vi "ScanAction.vi"(8 "error in (no error)":errorcluster caption="entrée d'erreur (pas d'erreur)", 9 "IndicePoint":i32, 10 "Dir":bool, 11 "Monospec In":refnum<class "Monospec50.lvclass"> caption="DNL_LabVIEW Object in") -> (0 "error out":errorcluster caption="sortie d'erreur", 2 "ScanParsOut":dbl[](array[numeric]), 3 "Monospec Out":refnum<class "Monospec50.lvclass"> caption="DNL_LabVIEW Object out")   [LabVIEW 2019, in "Monospec50.lvclass"]
uses:
  Monospec50.lvclass
  C:/Programmes Labview/LabScanV1A/DevicesClass/BaseDevice/BaseDevice.lvclass
  Monospec50.lvclass/Monospec50.ctl
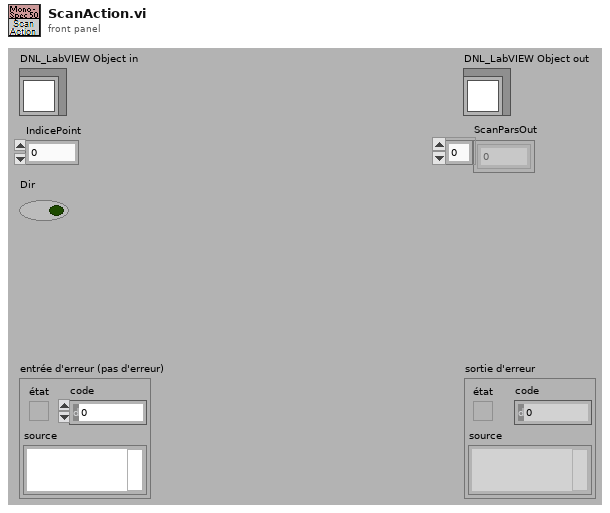
[diagram p1: front panel]
types:
  T1 = typedef "Monospec50.lvclass/Monospec50_Func.ctl" = enum16{"Position (nm)"}
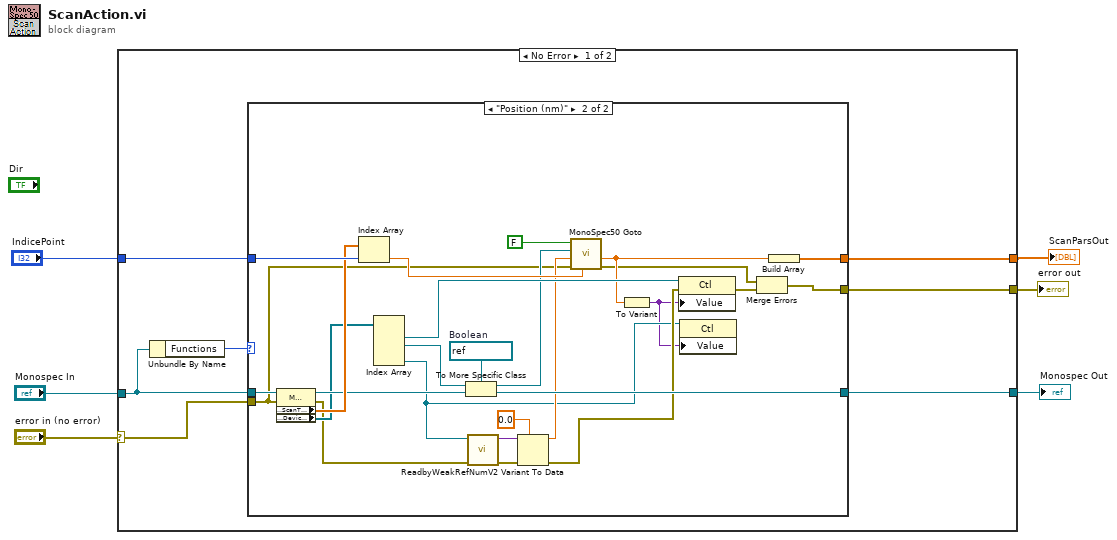
[diagram p0: block diagram]
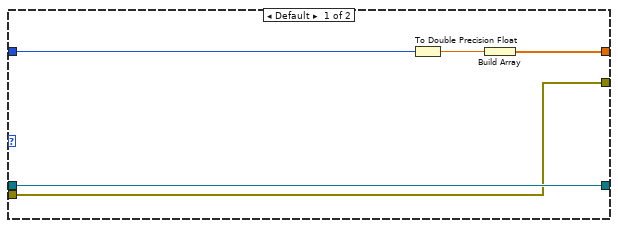
[diagram p2: hidden frame]
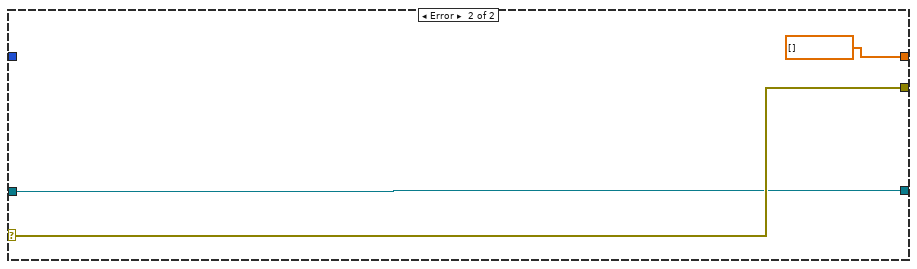
[diagram p3: hidden frame]
diagram:
  n1 = case shown="No Error" "error in (no error)" {
    selector: "error in (no error)" -> [w10 w46]
    tunnel: "Monospec In" -> [w11 w45]
    tunnel: [w9 dbl[] []] -> w1
    tunnel: [w8 w46] -> w4
    tunnel: [w7 w45] -> w3
    tunnel: "IndicePoint" -> [w12 _]
    frame No Error {
      n2 = Unbundle By Name(w11) -> ("Functions"=w13:T1)
      n3 = case shown="\"Position (nm)\"" w13 {
        tunnel: [w14 w43] -> w9
        tunnel: w12 -> [w18 w42]
        tunnel: [w16 w38] -> w7
        tunnel: w11 -> [w16 w40]
        tunnel: w10 -> [w15 w25]
        tunnel: [w15 w24] -> w8
        frame Default {
          n4 = To Double Precision Float(number=w18) -> (double precision float=w17:dbl)
          n5 = Build Array(w17) -> (w14:dbl[])
        }
        frame "Position (nm)" {
          w35 = refnum<vi> refnum  # Boolean
          n6 = property class="Monospec50.lvclass"(reference=w40, error in=w25) -> (reference out=w38:refnum<class "Monospec50.lvclass">, error out=w26:errorcluster, "Accessor:ScanTable"=w39:dbl[], "Accessor:DeviceCtrl"=w36:refnum<vi>[])
          n7 = Index Array(array=w39, index=w42) -> (element=w41:dbl)
          n8 = Index Array(array=w36) -> (element #1=w34:refnum<vi>, element #2=w32:refnum<vi>, element #4=w20:refnum<vi>)  [unwired: 4 in, 1 out]
          n9 = To More Specific Class(target class=w35, reference=w32) -> (specific class reference=w31:refnum<vi>)  [unwired: 1 in, 1 out]
          n10 = call <userlib>:"ReadbyWeakRefNumV2.vi"("error in"=w26, "Control Ref"=w20) -> ("error out"=w27:errorcluster, "Valeur"=w30:variant)  [unwired: 8 in]
          n11 = Variant To Data(error in=w27, type=0.0 ("PosAct"), Variant=w30) -> (data=w28:dbl, error out=w21:errorcluster)
          n12 = call <userlib>:"MonoSpec50 Goto.vi"("PosDem"=w41, "error in (no error)"=w25, "PosAct"=w28, "Moving Ref"=w31, "Ask Act Pos"=FALSE) -> ("error out"=w23:errorcluster, "PosAct Out"=w33:dbl)  [unwired: 3 in]
          n13 = To Variant(anything=w33) -> (Variant=w19:variant)
          n14 = property class="Ctl"(reference=w34, error in=w21, "Value"=w19) -> (error out=w22:errorcluster)  [unwired: 1 out]
          n15 = property class="Ctl"(reference=w20, "Value"=w19) -> ()  [unwired: 1 in, 2 out]
          n16 = Merge Errors(w23, w22) -> (w24:errorcluster)
          n17 = Build Array(w33) -> (w43:dbl[])
        }
      }
    }
    frame Error {
    }
  }
  "error out" <- w4
  "Monospec Out" <- w3
  "ScanParsOut" <- w1
